vi "Swap_CSG[].vi"(4 "Swap(T)":bool=TRUE, 6 "b":csg[](array[numeric]), 7 "a":csg[](array[numeric])) -> (1 "b":csg[](array[numeric]), 2 "a":csg[](array[numeric]))   [LabVIEW 2012]
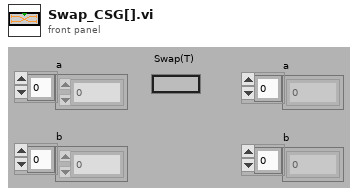
[diagram p1: front panel]
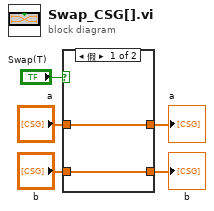
[diagram p0: block diagram]
diagram:
  n1 = case shown="假" "Swap(T)" {
    tunnel: "a" -> [w7 w9]
    tunnel: "b" -> [w6 w8]
    tunnel: [w7 w8] -> w2
    tunnel: [w6 w9] -> w1
    frame False {
    }
    frame True {
    }
  }
  "a" <- w2
  "b" <- w1
